vi "InitializePlayerBot.vi"(8 "error in (no error)":errorcluster, 10 "Player in":refnum<class "Player.lvclass">) -> (0 "error out":errorcluster, 1 "BotVIRefnum":T1, 2 "Player out":refnum<class "Player.lvclass">)   [LabVIEW 2015, in "TronviewGame.lvlib" / "Game.lvclass"]
uses:
  Game.lvclass
  Player/Player.lvclass
  BotVIRefnum.ctl
  TronviewGame.lvlib
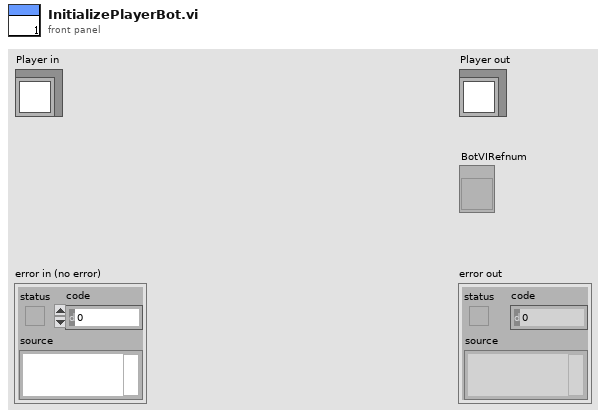
[diagram p1: front panel]
types:
  T1 = typedef "TronviewGame.lvlib/BotVIRefnum.ctl" = refnum<vi>
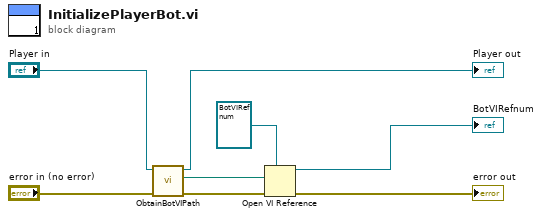
[diagram p0: block diagram]
diagram:
  n1 = call "ObtainBotVIPath.vi"("error in (no error)"="error in (no error)", "Player in"="Player in") -> ("error out"=w6:errorcluster, "BotPath"=w3:path, "Player out"=→"Player out":refnum<class "Player.lvclass">)  [unwired: 7 in]
  n2 = Open VI Reference(type specifier VI Refnum (for type only)=T1 refnum ("BotReference"), vi path=w3, error in (no error)=w6) -> (vi reference=→"BotVIRefnum":T1, error out=→"error out":errorcluster)  [unwired: 3 in]
